vi "Reports.Results V1 to JSON File With Data Files.vi"(6 "File Data Objs":T1[](array[typedef]), 7 "Temp Folder":path, 8 "error in (no error)":errorcluster, 9 "Test Result In":T2={"#attributes"={"Version"="MTE_1.0.0"}, "Station"={"Name"="", "PN"="", "SN"="", "Rev"="", "PC Name"="", "Location"="", "HW_Config"={"HW_Item"=[]}, "SW_Config"={"SW_Item"=[]}}, "Test Run"={"Operator"="", "Start Time"=timestamp(0 s since 1904-01-01), "Duration(s)"=0.0, "Mode"="", "Comment"="", "ProcessStep"=""}, "Test Sequence"={"Name"="", "Config"={"Config_Item"=[]}}, "UUTs"={"UUT"=[]}} {"UUTs"."UUT"."Measurements"."Measurement"."Status" items=["LOG", "PASS", "FAIL", "ERROR"]}, 10 "File Name":string, 11 "Folder":path) -> (0 "error out":errorcluster)   [LabVIEW 2018]
uses:
  Results/Result XML/TestResult.FullResultData.ctl
  Results/Result XML/TestResult.Station Info.ctl
  Results/Result XML/TestResult.HW Item.ctl
  Results/Result XML/TestResult.SW Item.ctl
  Results/Result XML/TestResult.Test Run Info.ctl
  Results/Result XML/TestResult.Test Info.ctl
  Results/Result XML/TestResult.UUT Result.ctl
  Results/Result XML/TestResult.Symptom.ctl
  Results/Result XML/TestResult.Symptom.State.ctl
  Results/Result.Measurement Item.ctl
  Results/Result.Measurement and Attribute Item Status.ctl
  Results/Result XML/TestResult.UUTInfo.ctl
  Report.Result FileDataObject.ctl
  <vilib>/KATE/Files/File Utils.lvlib
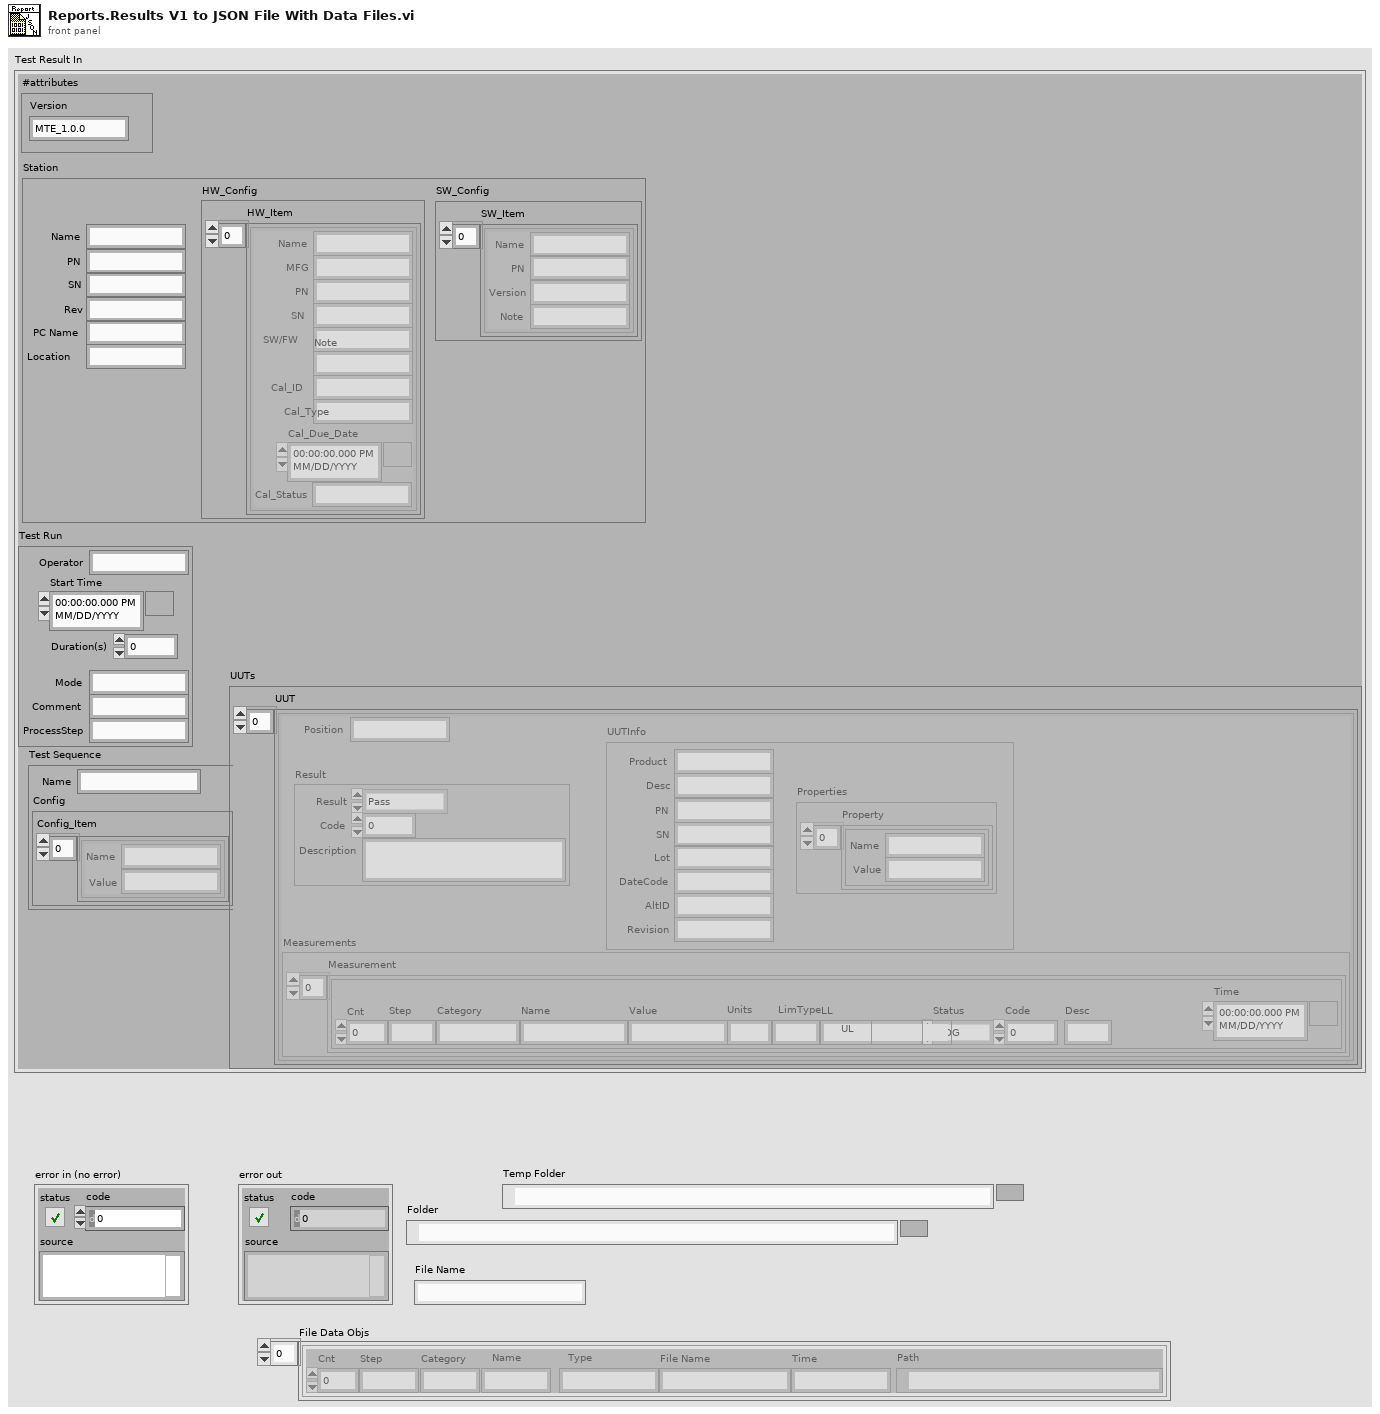
[diagram p1: front panel]
types:
  T1 = typedef "Report.Result FileDataObject.ctl" = cluster{"Cnt":i32, "Step":string, "Category":string, "Name":string, "Type":string, "File Name":string, "Time":string, "Path":path}
  T2 = typedef "TestResult.FullResultData.ctl" = cluster{"#attributes":cluster{"Version":string}, "Station":T3, "Test Run":T6, "Test Sequence":T7, "UUTs":cluster{"UUT":T8[]}}
  T3 = typedef "TestResult.Station Info.ctl" = cluster{"Name":string, "PN":string, "SN":string, "Rev":string, "PC Name":string, "Location":string, "HW_Config":cluster{"HW_Item":T4[]}, "SW_Config":cluster{"SW_Item":T5[]}}
  T4 = typedef "TestResult.HW Item.ctl" = cluster{"Name":string, "MFG":string, "PN":string, "SN":string, "SW/FW":string, "Note":string, "Cal_ID":string, "Cal_Type":string, "Cal_Due_Date":timestamp, "Cal_Status":string}
  T5 = typedef "TestResult.SW Item.ctl" = cluster{"Name":string, "PN":string, "Version":string, "Note":string}
  T6 = typedef "TestResult.Test Run Info.ctl" = cluster{"Operator":string, "Start Time":timestamp, "Duration(s)":dbl, "Mode":string, "Comment":string, "ProcessStep":string}
  T7 = typedef "TestResult.Test Info.ctl" = cluster{"Name":string, "Config":cluster{"Config_Item":cluster{"Name":string, "Value":string}[]}}
  T8 = typedef "TestResult.UUT Result.ctl" = cluster{"Position":string, "Result":T9, "Measurements":cluster{"Measurement":T11[]}, "UUTInfo":T13}
  T9 = typedef "TestResult.Symptom.ctl" = cluster{"Result":T10, "Code":i32, "Description":string}
  T10 = typedef "TestResult.Symptom.State.ctl" = enum16{"Pass", "Fail", "Error", "Aborted", "Completed", "Logged"}
  T11 = typedef "Result.Measurement Item.ctl" = cluster{"Cnt":i32, "Step":string, "Category":string, "Name":string, "Value":string, "Units":string, "LimType":string, "LL":string, "UL":string, "Status":T12, "Code":i32, "Desc":string, "Time":timestamp}
  T12 = typedef "Result.Measurement and Attribute Item Status.ctl" = i32
  T13 = typedef "TestResult.UUTInfo.ctl" = cluster{"Product":string, "Desc":string, "PN":string, "SN":string, "Lot":string, "DateCode":string, "AltID":string, "Revision":string, "Properties":cluster{"Property":cluster{"Name":string, "Value":string}[]}}
  T14 = typedef "Report.Result Data JSON V2.0.0.ctl" = cluster{"Type":string, "Version":string, "TestEvent":T15, "UUTInfo":T17, "Station":T18, "TestSequence":T19, "ResultData":T20[], "DataObjs":T21[]}
  T15 = typedef "Report.Result Test Event.ctl" = cluster{"ProcessStep":string, "StartTime":string, "EndTime":string, "Mode":string, "Operator":string, "Comment":string, "Result":T16}
  T16 = typedef "Report.Result State.ctl" = cluster{"State":string, "Code":i32, "Desc":string, "Details":string}
  T17 = typedef "Report.Result UUTInfo.ctl" = cluster{"Product":string, "Description":string, "PN":string, "SN":string, "LotNumber":string, "DateCode":string, "AltID":string, "Revision":string, "Properties":cluster{"Name":string, "Value":string}[]}
  T18 = typedef "Report.Result Test Station.ctl" = cluster{"Name":string, "Location":string, "ConfigID":string, "PCName":string, "Slot":string}
  T19 = typedef "Report.Result Test Sequence.ctl" = cluster{"Name":string, "Setup":cluster{"Name":string, "Value":string}[]}
  T20 = typedef "Report.Result Measurement JSON Safe.ctl" = cluster{"Cnt":i32, "Step":string, "Category":string, "Name":string, "Value":string, "Units":string, "LimType":string, "LL":string, "UL":string, "Time":string, "Result":T16}
  T21 = typedef "Report.Result DataObject.ctl" = cluster{"Cnt":i32, "Step":string, "Category":string, "Name":string, "Type":string, "FileName":string, "Time":string}
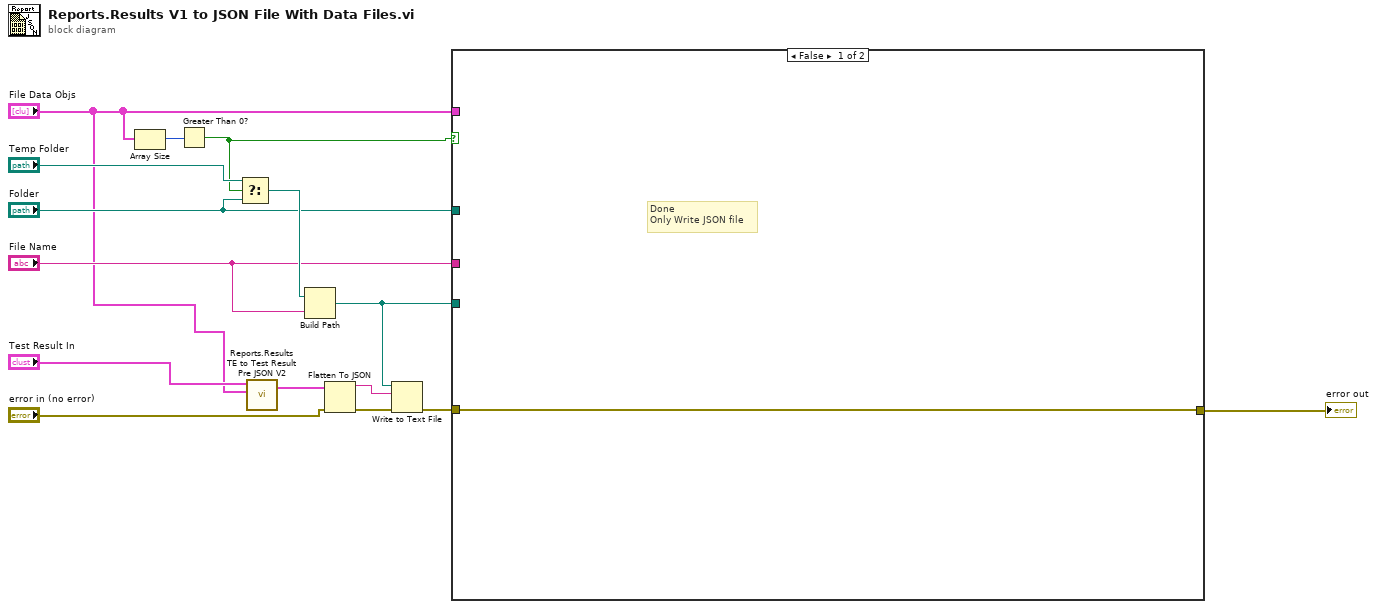
[diagram p0: block diagram]
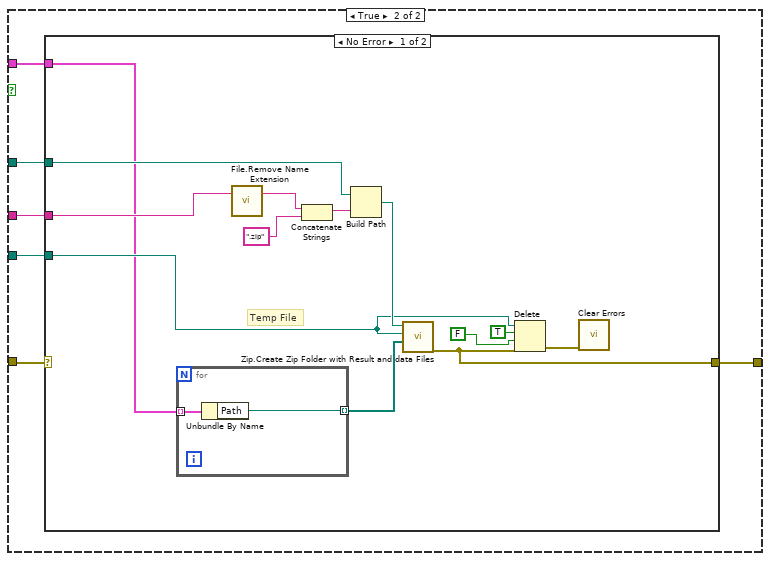
[diagram p2: hidden frame]
diagram:
  n1 = Array Size(array="File Data Objs") -> (size(s)=w10:i32)
  n2 = Greater Than 0?(x=w10) -> (x > 0?=w7:bool)
  n3 = Select(t="Temp Folder", s=w7, f="Folder") -> (s? t:f=w8:path)
  n4 = call "Reports.Results TE to Test Result Pre JSON V2.vi"("File Data Objs"="File Data Objs", "Test Result In"="Test Result In") -> ("Test Result V2"=w13:T14)  [unwired: 3 in]
  n5 = Build Path(base path=w8, name or relative path="File Name") -> (appended path=w5:path)
  n6 = Flatten To JSON(anything=w13, error in (no error)="error in (no error)") -> (JSON string=w14:string, 11:w12:errorcluster)  [unwired: 1 in]
  n7 = Write to Text File(file (use dialog)=w5, text=w14, error in=w12) -> (error out=w6:errorcluster)  [unwired: 1 in, 2 out]
  n8 = case shown="False" w7 {
    tunnel: w6 -> [w16 w22]
    tunnel: w5 -> [_ w17]
    tunnel: [w16 w21] -> w4
    tunnel: "File Name" -> [_ w20]
    tunnel: "Folder" -> [_ w19]
    tunnel: "File Data Objs" -> [_ w18]
    frame False {
      # "Done\nOnly Write JSON file"
    }
    frame True {
      n9 = case shown="No Error" w22 {
        selector: w22 -> [_ w38]
        tunnel: [w26 w38] -> w21
        tunnel: w20 -> [w29 _]
        tunnel: w19 -> [w28 _]
        tunnel: w18 -> [w24 _]
        tunnel: w17 -> [w27 _]
        frame No Error {
          # "Temp File"
          n10 = for {
            tunnel: w24 -> [w37] mode=indexing
            tunnel: [w36] -> w23 mode=indexing
            n11 = Unbundle By Name(w37) -> ("Path"=w36:path)
          }
          n12 = call <vilib>:"File.Remove Name Extension.vi"("File Name"=w29) -> ("Name Less Ext"=w33:string)  [unwired: 1 in, 1 out]
          n13 = Concatenate Strings(w33, ".zip" ("string")) -> (w34:string)
          n14 = Build Path(base path=w28, name or relative path=w34) -> (appended path=w35:path)
          n15 = call "Zip.Create Zip Folder with Result and data Files.vi"("Data Files"=w23, "Result File"=w27, "Output Zip File"=w35) -> ("error out"=w26:errorcluster)  [unwired: 8 in]
          n16 = Delete(path (use dialog)=w27, entire hierarchy (F)=TRUE, confirm (F)=FALSE, error in=w26) -> (error out=w25:errorcluster)  [unwired: 1 in, 2 out]
          n17 = call <vilib>:"Clear Errors.vi"("error in (no error)"=w25) -> ()  [unwired: 5 in, 2 out]
        }
        frame Error {
        }
      }
    }
  }
  "error out" <- w4
